vi "Progress Window.vi"(9 "Stop":refnum<data-value>, 10 "Progress":refnum<data-value>, 11 "Status String":refnum<data-value>) -> ()   [LabVIEW 2017, in "Build Automation.lvlib"]
uses:
  Build Automation.lvlib
panel:
  in  "Cancel":bool
  out "Status Message":string
  out "Progress":dbl(slide) scale=0.0..100.0 scale format="%.1f"
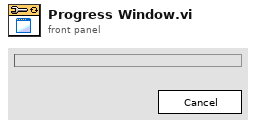
[diagram p1: front panel]
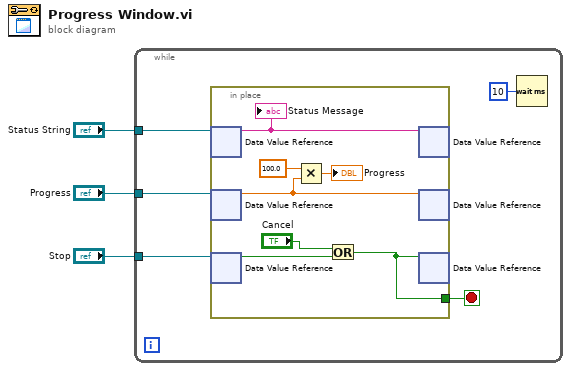
[diagram p0: block diagram]
diagram:
  n1 = while {
    tunnel: "Status String" -> [w7]
    tunnel: "Stop" -> [w6]
    tunnel: "Progress" -> [w4]
    stop <- w5 stop-if-true
    n2 = in-place {
      in-place-border: [w9] -> w5
      n3 = in-place-dvr #1(w7) -> (w15:string)  [unwired: 1 out]
      "Status Message" <- w15
      n4 = in-place-dvr #2(w4) -> (w13:dbl)  [unwired: 1 out]
      n5 = in-place-dvr #3(w6) -> (w11:bool)  [unwired: 1 out]
      n6 = Multiply(x=100.0, y=w13) -> (x*y=→"Progress":dbl)
      n7 = Or(x="Cancel", y=w11) -> (x .or. y?=w9:bool)
      n8 = in-place-dvr #1(w15) -> ()  [unwired: 2 out]
      n9 = in-place-dvr #2(w13) -> ()  [unwired: 2 out]
      n10 = in-place-dvr #3(w9) -> ()  [unwired: 2 out]
    }
    n11 = Wait (ms)(milliseconds to wait=u32 10) -> ()  [unwired: 1 out]
  }
